vi "Initialize RT Variables.vi"() -> (0 "error out":errorcluster, 1 "Sync Guard Data":fxp<+/-,38,12>[](array[numeric]) format="%.9g", 2 "Data Size":u32, 3 "FPGA Refnum out":T1)   [LabVIEW 2022 SP3]
doc: "Author: Scott Hannahs <sth@magnet.fsu.edu>\nCopyright 2018 Florida State University, All rights reserved."
uses:
  RT Controls/FPGA SCH Digitizer Ref.ctl
  <vilib>/userDefined/Silver/nirio_resource_slv.ctl
  RT Host Globals.vi
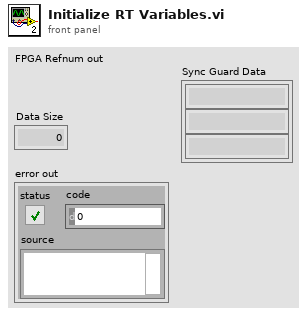
[diagram p1: front panel]
types:
  T1 = typedef "FPGA SCH Digitizer Ref.ctl" = refnum<k20>
  T2 = typedef "nirio_resource_slv.ctl" = tag
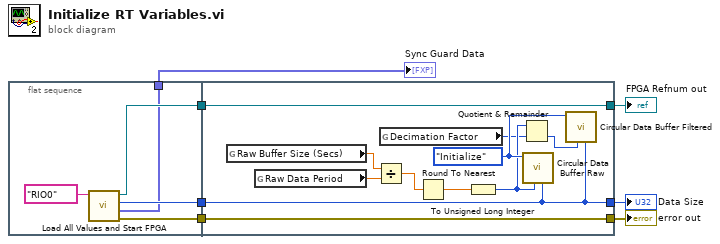
[diagram p0: block diagram]
diagram:
  n1 = flat-sequence {
    tunnel: [w12] -> w7
    tunnel: [w10] -> w6
    tunnel: [w11] -> w5
    tunnel: [w8] -> w3
    tunnel: w7 -> [w14]
    tunnel: w6 -> [w22]
    tunnel: w5 -> [w13]
    tunnel: [w22] -> w4
    tunnel: [w14] -> w2
    tunnel: [w13] -> w1
    frame #0 {
      n2 = call "Load All Values and Start FPGA.vi"("Resource name"=T2 "RIO0" ("resource name")) -> ("error out"=w11:errorcluster, "Sync Guard Data"=w8:fxp<+/-,38,12>[], "Data Size"=w10:u32, "FPGA Refnum out"=w12:T1)  [unwired: 7 in]
    }
    frame #1 {
      w23 = enum16{"Initialize", "Write", "Read", "Clear"}."Initialize" ("Enum")
      n3 = global read "RT Host Globals.vi" "Raw Buffer Size (Secs)"() -> (w21:dbl)
      n4 = global read "RT Host Globals.vi" "Raw Data Period"() -> (w20:dbl)
      n5 = Divide(x=w21, y=w20) -> (x/y=w19:dbl)
      n6 = global read "RT Host Globals.vi" "Decimation Factor"() -> (w16:u32)
      n7 = Round To Nearest(number=w19) -> (nearest integer value=w18:dbl)
      n8 = To Unsigned Long Integer(number=w18) -> (unsigned 32bit integer=w17:u32)
      n9 = Quotient & Remainder(x=w17, y=w16) -> (floor(x/y)=w15:u32)  [unwired: 1 out]
      n10 = call "Circular Data Buffer Raw.vi"("Row Size"=w22, "Buffer Size"=w17, "Enum"=w23) -> ()  [unwired: 6 in, 3 out]
      n11 = call "Circular Data Buffer Filtered.vi"("Row Size"=w22, "Buffer Size"=w15, "Action"=w23) -> ()  [unwired: 6 in, 3 out]
    }
  }
  "FPGA Refnum out" <- w2
  "error out" <- w1
  "Data Size" <- w4
  "Sync Guard Data" <- w3
